vi "Save_Displacement_in_Array(Track)-1.vi"(2 "[IN] Index for Collect":i32, 3 "[IN] Collecting Array":dbl[](array[numeric]), 4 "[IN] Index of displ":i32, 5 "[IN]Source Array":dbl[](array[numeric])) -> (0 "[OUT] Finish Index for Collect":i32, 1 "[OUT] Collecting Array":dbl[](array[numeric]))   [LabVIEW 2017]
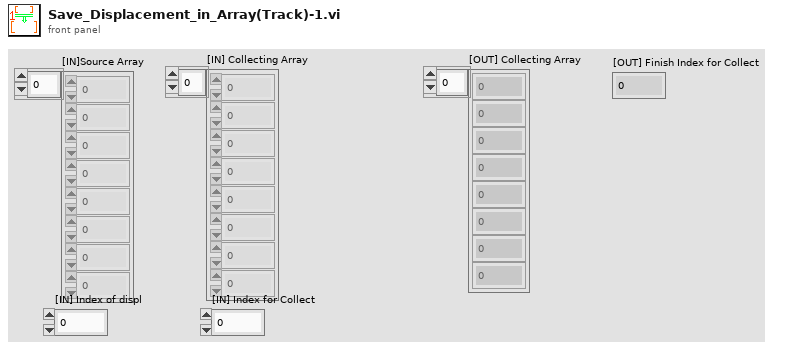
[diagram p1: front panel]
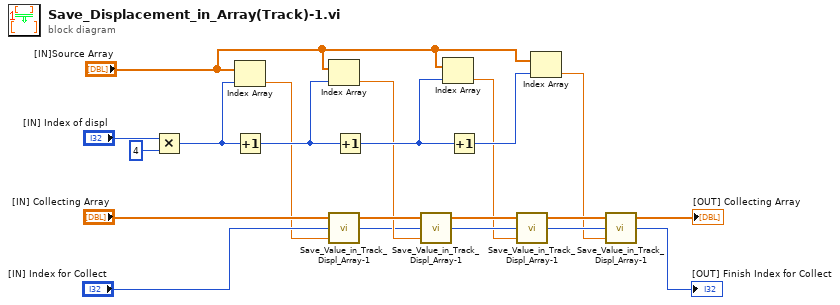
[diagram p0: block diagram]
diagram:
  n1 = Multiply(x="[IN] Index of displ", y=4) -> (x*y=w15:i32)
  n2 = Index Array(array="[IN]Source Array", index=w15) -> (element=w12:dbl)
  n3 = Increment(x=w15) -> (x+1=w21:i32)
  n4 = Index Array(array="[IN]Source Array", index=w21) -> (element=w10:dbl)
  n5 = call "Save_Value_in_Track_Displ_Array-1.vi"("[IN] Value"=w12, "[IN] Index"="[IN] Index for Collect", "[IN] Empty tracks\nfor points saving"="[IN] Collecting Array") -> ("[OUT] Index ++"=w9:i32, "[OUT Track with saved value"=w11:dbl[])  [unwired: 1 in]
  n6 = Increment(x=w21) -> (x+1=w20:i32)
  n7 = call "Save_Value_in_Track_Displ_Array-1.vi"("[IN] Value"=w10, "[IN] Index"=w9, "[IN] Empty tracks\nfor points saving"=w11) -> ("[OUT] Index ++"=w7:i32, "[OUT Track with saved value"=w8:dbl[])  [unwired: 1 in]
  n8 = Index Array(array="[IN]Source Array", index=w20) -> (element=w6:dbl)
  n9 = Increment(x=w20) -> (x+1=w19:i32)
  n10 = call "Save_Value_in_Track_Displ_Array-1.vi"("[IN] Value"=w6, "[IN] Index"=w7, "[IN] Empty tracks\nfor points saving"=w8) -> ("[OUT] Index ++"=w4:i32, "[OUT Track with saved value"=w5:dbl[])  [unwired: 1 in]
  n11 = Index Array(array="[IN]Source Array", index=w19) -> (element=w2:dbl)
  n12 = call "Save_Value_in_Track_Displ_Array-1.vi"("[IN] Value"=w2, "[IN] Index"=w4, "[IN] Empty tracks\nfor points saving"=w5) -> ("[OUT] Index ++"=→"[OUT] Finish Index for Collect":i32, "[OUT Track with saved value"=→"[OUT] Collecting Array":dbl[])  [unwired: 1 in]
